vi "ADS Detect.vi"(5 "Height":u32, 6 "Pixel Size (Bytes)":i32, 7 "Width":u32, 8 "error in (no error)":errorcluster, 9 "LineWidth(Pixels)":i32, 10 "Pixel Pointer in":u64, 11 "ref in":u64) -> (0 "error out":errorcluster, 2 "return type":i32, 3 "ref out":u64)   [LabVIEW 2024]
uses:
  dependencies_dll_release/TCV_Lib.dll
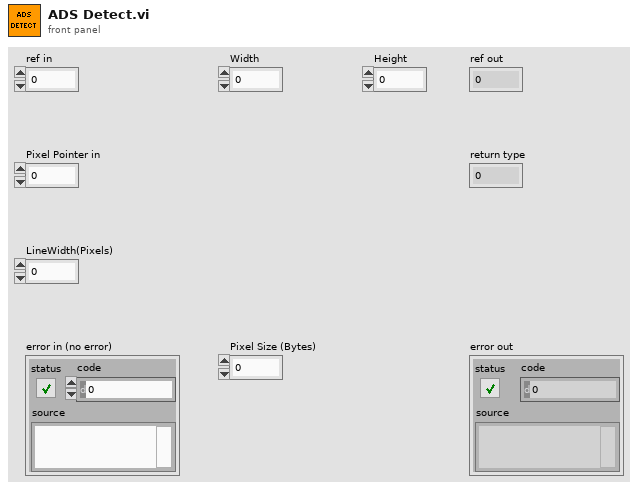
[diagram p1: front panel]
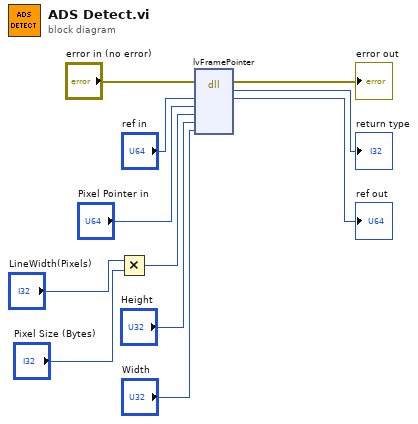
[diagram p0: block diagram]
diagram:
  n1 = Multiply(x="LineWidth(Pixels)", y="Pixel Size (Bytes)") -> (x*y=w6:i32)
  n2 = dll-call lib="D:/labviewTestTCVdll/TransformCV-LabVIEW/Test/dependencies_dll_release/TCV_Lib.dll" fn="lvFramePointer"(error in="error in (no error)", "ref"="ref in", "ImagePointer"="Pixel Pointer in", "Linewidth"=w6, "h"="Height", "w"="Width") -> (error out=→"error out":errorcluster, "return"=→"return type":i32, "ref"=→"ref out":u64)  [unwired: 6 in, 1 out]
